vi "Register Address to Synchronization Register.vi"(11 "address":u16) -> (3 "register":T1)   [LabVIEW 2014, in "ni579x Synchronization v2 FPGA.lvlib"]
uses:
  <instrlib>/ni579x/Synchronization/v2/FPGA/ni579x Synchronization v2 FPGA.lvlib
  <instrlib>/ni579x/Synchronization/v2/Shared/ni579x Synchronization Register Addresses.ctl
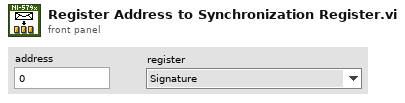
[diagram p1: front panel]
types:
  T1 = typedef "ni579x Synchronization Register Addresses.ctl" = enum16{"Signature", "Current Version", "Oldest Compatible Version", "Scratch Register", "sync.master", "sync.meas.enable", "sync.meas.ready", "sync.meas.arm", "sync.meas.valid", "sync.meas.value", "sync.cptr.adjust", "sync.cptr.period", "sync.meas.oversample factor"}
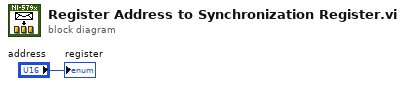
[diagram p0: block diagram]
diagram:
  "register" <- "address"
